vi "floatToString.vi"(11 "Numeric":dbl) -> (3 "String":string)   [LabVIEW 2011]
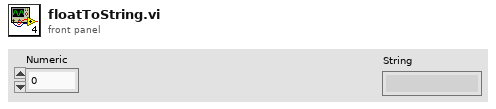
[diagram p1: front panel]
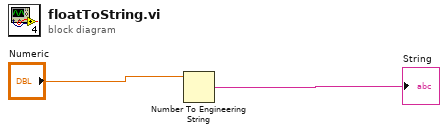
[diagram p0: block diagram]
diagram:
  n1 = Number To Engineering String(4:"Numeric") -> (0:→"String":string)  [unwired: 3 in]
